vi "Light_Sheet.vi"() -> ()   [LabVIEW 2011]
panel:
  out "Error":bool[](array[boolean])
  in  "Channel Name":string="Lanta:Laser:Control"
  in  "Port Name":string="hydrosonic"
  in  "DMX Start channel no.":u8=1
  in  "Z-Axis Rotation":u16(ring)=190 items=["Manual"=50, "Auto"=190]
  in  "X-Axis Rotation":u16(ring)=170 items=["Manual"=50, "Auto"=170]
  in  "Y-Axis Rotation":u16(ring)=170 items=["Manual"=50, "Auto"=170]
  in  "Zoom":u16(ring)=10 items=["None"=10, "Manual"=50, "Auto Out"=100, "Auto In"=155, "Auto 2 Way"=220]
  in  "Vertical Motion":u16(ring)=170 items=["Manual"=10, "Auto Down/Up"=170, "Auto Up/Down"=205, "Auto 2 Way"=230]
  in  "Horizontal Motion":u16(ring)=195 items=["Manual"=10, "Auto 1 Way"=195, "Auto 2 Way"=230]
  in  "Brightness":u16(ring)=10 items=["Normal"=10, "Bright"=80]
  in  "Strobe":u16(ring)=195 items=["Least 1"=10, "2"=50, "3"=80, "4"=150, "5"=195, "6"=205, "7"=212, "8"=218, "Most 9"=230]
  in  "Pattern":u16(ring)=80 items=["Static"=10, "Moving"=80, "Animation"=230]
  in  "Operating Mode":u16(ring)=170 items=["Off"=10, "Manual"=212, "Auto Run"=170, "Sound Active"=80]
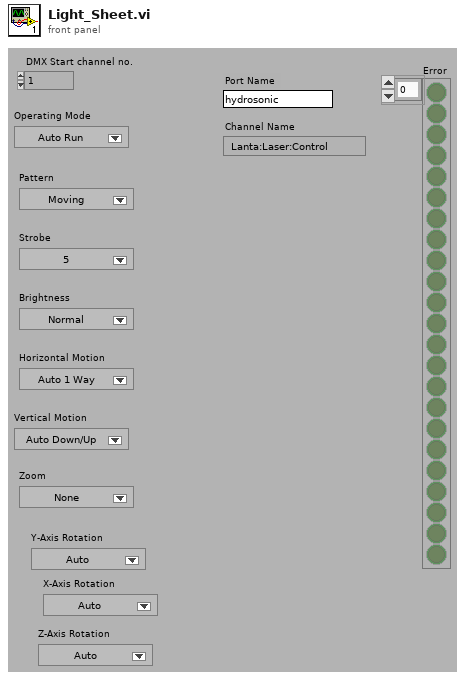
[diagram p1: front panel]
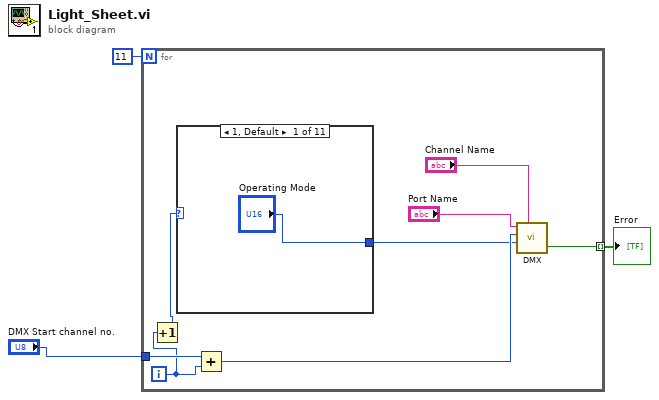
[diagram p0: block diagram]
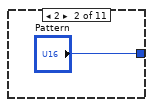
[diagram p2: hidden frame]
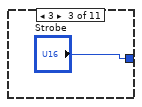
[diagram p3: hidden frame]
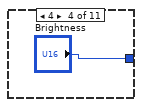
[diagram p4: hidden frame]
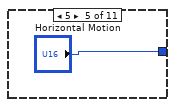
[diagram p5: hidden frame]
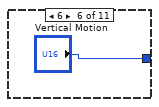
[diagram p6: hidden frame]
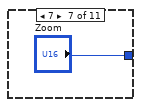
[diagram p7: hidden frame]
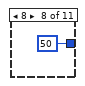
[diagram p8: hidden frame]
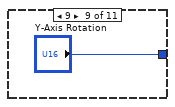
[diagram p9: hidden frame]
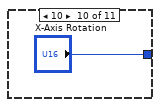
[diagram p10: hidden frame]
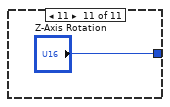
[diagram p11: hidden frame]
diagram:
  n1 = for {
    N: 11 -> [_]
    tunnel: "DMX Start channel no." -> [w9]
    tunnel: [w4] -> w1 mode=indexing
    i -> [w7]
    n2 = Increment(x=w7) -> (x+1=w6:i32)
    n3 = case shown="1, Default" w6 {
      tunnel: ["Operating Mode" "Pattern" "Strobe" "Brightness" "Horizontal Motion" "Vertical Motion" "Zoom" u16 50 ("Z-Axis Rotation") "Y-Axis Rotation" "X-Axis Rotation" "Z-Axis Rotation"] -> w5
      frame 1, Default {
      }
      frame 2 {
      }
      frame 3 {
      }
      frame 4 {
      }
      frame 5 {
      }
      frame 6 {
      }
      frame 7 {
      }
      frame 8 {
      }
      frame 9 {
      }
      frame 10 {
      }
      frame 11 {
      }
    }
    n4 = Add(x=w9, y=w7) -> (x+y=w8:i32)
    n5 = call "DMX.vi"("Port Name"="Port Name", "DMX channel no."=w8, "Set value:"=w5, "Channel Name"="Channel Name") -> ("error"=w4:bool)  [unwired: 1 in, 1 out]
  }
  "Error" <- w1
